vi "Rx Message to Transfer Handle - BC.vi"(8 "error in":errorcluster, 9 "message":T2={"name"="", "message type"="BC to RT", "endpoint Tx"={"terminal address"=0, "subaddress"=0}, "endpoint Rx"={"terminal address"=0, "subaddress"=0}, "create timestamp channel"=FALSE, "mode code"=0, "number of words"=0, "parameters"=[]}, 11 "bus controller handle":u64) -> (0 "error out":errorcluster, 2 "valid?":bool, 3 "Rx read info":T1)   [LabVIEW 2023, in "Ballard MIL-STD-1553 Engine Support.lvlib" / "Custom Device.lvlib"]
uses:
  Custom Device.lvlib
  Shared/Message Definition.ctl
  Shared/Message Type.ctl
  Shared/Terminal Endpoint.ctl
  Shared/Address.ctl
  Shared/Parameter Definition.ctl
  Shared/Rx Read Info.ctl
  Scripting/Constants.vi
  <instrlib>/BTI1553Lib/BTI1553LV.lvlib
  Scripting/Ballard MIL-STD-1553 Scripting.lvlib
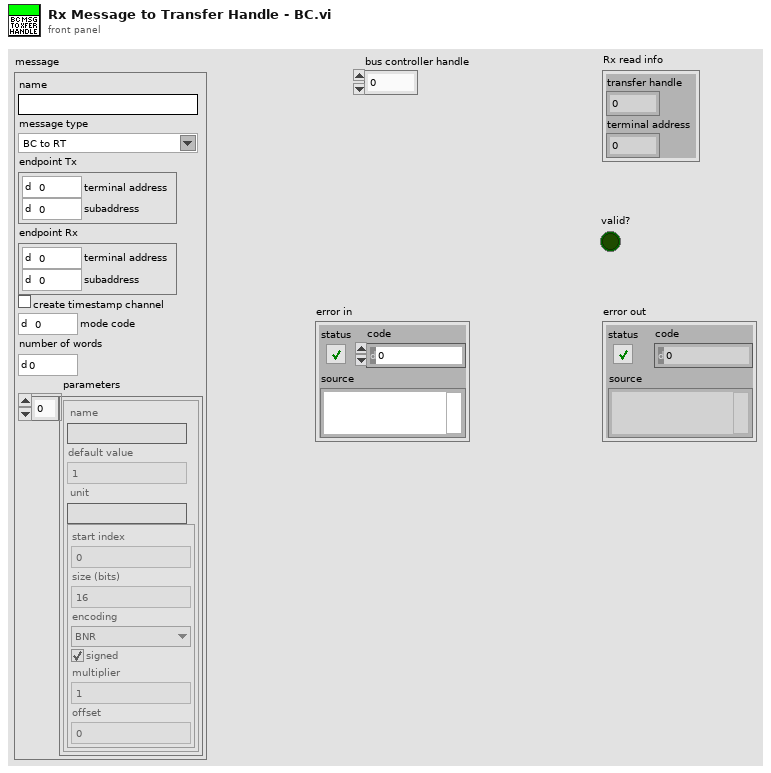
[diagram p1: front panel]
types:
  T1 = typedef "Rx Read Info.ctl" = cluster{"transfer handle":u64, "terminal address":u16}
  T2 = typedef "Message Definition.ctl" = cluster{"name":string, "message type":T3, "endpoint Tx":T4, "endpoint Rx":T4, "create timestamp channel":bool, "mode code":u16, "number of words":u16, "parameters":cluster{"name":string, "default value":dbl, "unit":string, "parameter definition":T6}[]}
  T3 = typedef "Message Type.ctl" = string
  T4 = typedef "Terminal Endpoint.ctl" = cluster{"terminal address":T5, "subaddress":T5}
  T5 = typedef "Address.ctl" = u16
  T6 = typedef "Parameter Definition.ctl" = cluster{"start index":i32, "size (bits)":i32, "encoding":enum16{"BNR", "BCD", "Discrete"}, "signed":bool, "multiplier":dbl, "offset":dbl}
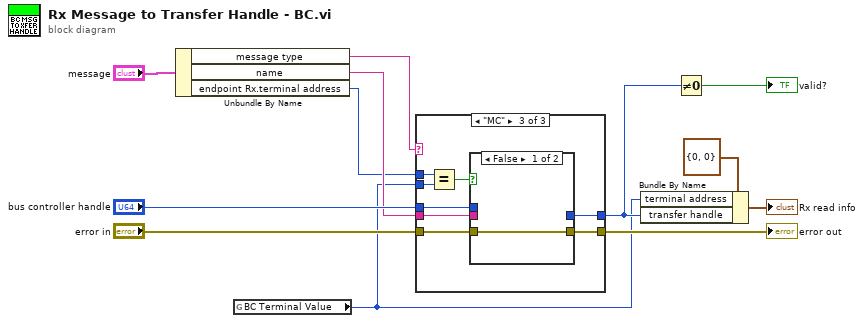
[diagram p0: block diagram]
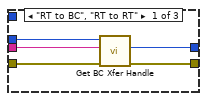
[diagram p2: hidden frame]
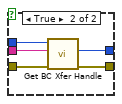
[diagram p4: hidden frame]
diagram:
  n1 = Unbundle By Name("message") -> ("message type"=w2:T3, "name"=w4:string, "endpoint Rx.terminal address"=w3:T5)
  n2 = global read "Constants.vi" "BC Terminal Value"() -> (w1:u16)
  n3 = case shown="\"MC\"" w2 {
    tunnel: "error in" -> [w17 w18 w26]
    tunnel: [w16 w18 w25] -> w10
    tunnel: "bus controller handle" -> [w13 _ w24]
    tunnel: [w15 _ w23] -> w5
    tunnel: w4 -> [w14 _ w22]
    tunnel: w3 -> [_ _ w20]
    tunnel: w1 -> [_ _ w19]
    frame "RT to BC", "RT to RT" {
      n4 = call <instrlib>:"Get BC Xfer Handle.vi"("error in (no error)"=w17, "bc transfer name"=w14, "bus controller handle in"=w13) -> ("error out"=w16:errorcluster, "bc transfer handle out"=w15:u64)  [unwired: 6 in, 1 out]
    }
    frame "BC to RT", Default {
    }
    frame "MC" {
      n5 = Equal?(x=w20, y=w19) -> (x = y?=w21:bool)
      n6 = case shown="False" w21 {
        tunnel: w26 -> [w27 w32]
        tunnel: [w27 w31] -> w25
        tunnel: w24 -> [_ w30]
        tunnel: [_ w29] -> w23
        tunnel: w22 -> [_ w28]
        frame False {
        }
        frame True {
          n7 = call <instrlib>:"Get BC Xfer Handle.vi"("error in (no error)"=w32, "bc transfer name"=w28, "bus controller handle in"=w30) -> ("error out"=w31:errorcluster, "bc transfer handle out"=w29:u64)  [unwired: 6 in, 1 out]
        }
      }
    }
  }
  "error out" <- w10
  n8 = Bundle By Name(cluster=T1 {"transfer handle"=0, "terminal address"=0} ("Rx read info"), "terminal address"=w1, "transfer handle"=w5) -> (→"Rx read info":T1)
  n9 = Not Equal To 0?(x=w5) -> (x != 0?=→"valid?":bool)
